vi "COM Error Checker.vi"(8 "error in (no error)":errorcluster, 10 "Command":string, 11 "Response":string) -> (0 "error out":errorcluster, 3 "String":string)   [LabVIEW 2019, in "KH7008.lvlib"]
uses:
  KH7008.lvlib
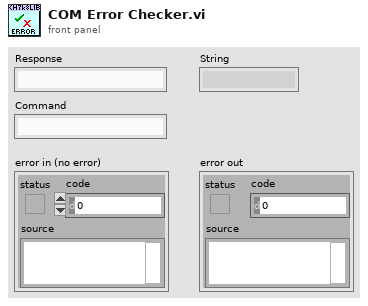
[diagram p1: front panel]
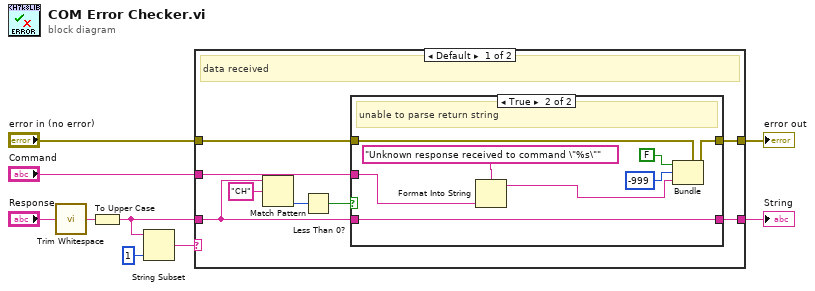
[diagram p0: block diagram]
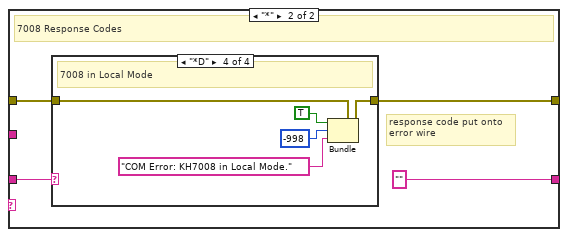
[diagram p3: hidden frame]
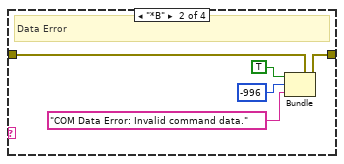
[diagram p5: hidden frame]
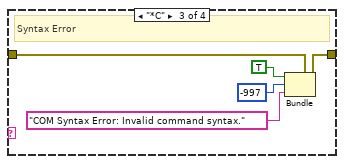
[diagram p6: hidden frame]
diagram:
  n1 = call <vilib>:"Trim Whitespace.vi"("string"="Response") -> ("trimmed string"=w4:string)  [unwired: 1 in]
  n2 = To Upper Case(1:w4) -> (0:w2:string)
  n3 = String Subset(string=w2, length (rest)=1 ("length (rest)")) -> (substring=w5:string)  [unwired: 1 in]
  n4 = case shown="Default" w5 {
    tunnel: [w14 w31] -> w9
    tunnel: "error in (no error)" -> [w15 w30]
    tunnel: w2 -> [w12 w29]
    tunnel: [w11 "" ("trimmed string")] -> w3
    tunnel: "Command" -> [w10 _]
    frame Default {
      # "data received"
      n5 = Match Pattern(string=w12, regular expression="CH") -> (offset past match=w16:i32)  [unwired: 1 in, 3 out]
      n6 = Less Than 0?(x=w16) -> (x < 0?=w13:bool)
      n7 = case shown="True" w13 {
        tunnel: w15 -> [w19 w25]
        tunnel: [w19 w24] -> w14
        tunnel: w12 -> [w18 w23]
        tunnel: [w18 w23] -> w11
        tunnel: w10 -> [_ w21]
        frame False {
          # "Data Ok, No errors"
        }
        frame True {
          # "unable to parse return string"
          n8 = Format Into String(format string="Unknown response received to command \"%s\"" ("source"), w21) -> (resulting string=w20:string)  [unwired: 2 in, 1 out]
          n9 = Bundle(cluster=w25, "status"=FALSE, "code"=-999, "source"=w20) -> (w24:errorcluster)
        }
      }
    }
    frame "*" {
      # "response code put onto\nerror wire"
      # "7008 Response Codes"
      n10 = case shown="\"*D\"" w29 {
        tunnel: w30 -> [w32 w37 w42 w47]
        tunnel: [w32 w33 w38 w43] -> w31
        frame "*A", Default {
          # "Data Ok, No errors"
        }
        frame "*B" {
          # "Data Error"
          n11 = Bundle(cluster=w37, "status"=TRUE, "code"=-996, "source"="COM Data Error: Invalid command data.") -> (w33:errorcluster)
        }
        frame "*C" {
          # "Syntax Error"
          n12 = Bundle(cluster=w42, "status"=TRUE, "code"=-997, "source"="COM Syntax Error: Invalid command syntax.") -> (w38:errorcluster)
        }
        frame "*D" {
          # "7008 in Local Mode"
          n13 = Bundle(cluster=w47, "status"=TRUE, "code"=-998, "source"="COM Error: KH7008 in Local Mode.") -> (w43:errorcluster)
        }
      }
    }
  }
  "String" <- w3
  "error out" <- w9
